vi "Update Vision Data.vi"(8 "error in (no error)":errorcluster, 10 "unsigned byte array":u8[](array[numeric]), 11 "Vision in":refnum<class "Vision.lvclass">) -> (0 "error out":errorcluster, 3 "Vision out":refnum<class "Vision.lvclass">)   [LabVIEW 2022 SP3, in "Vision.lvlib" / "Vision.lvclass"]
uses:
  Vision.lvclass
  Vision.lvclass/Vision.ctl
  Old vision/Decode SSL and Refree Wrapper Package Folder/Varint Decoder uint32.vi
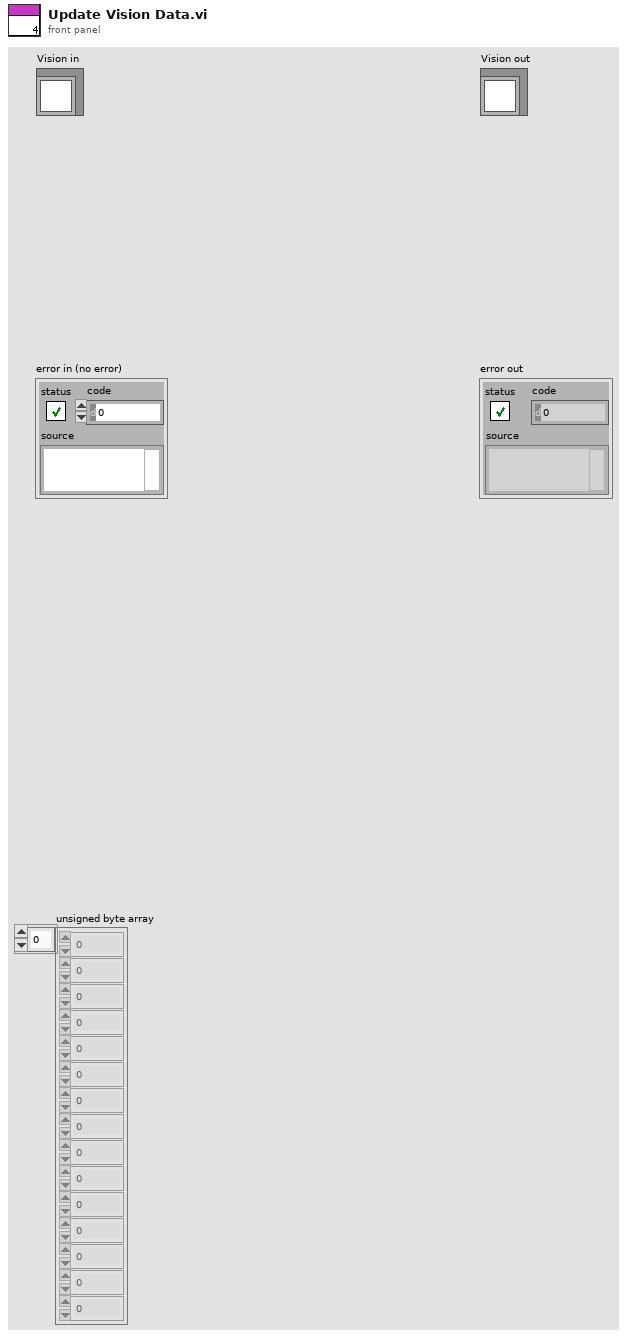
[diagram p1: front panel]
types:
  T1 = typedef "SSL Detection Frame.ctl" = cluster{"frame_number":u32, "t_capture":dbl, "t_sent":dbl, "camera_id":u32, "robots_yellow":T2[], "robots_blue":T2[], "balls":T4[], "Valid":bool, "Time Stamp":timestamp, "New":bool, "Initialized":bool}
  T2 = typedef "SSL Detection Robot.ctl" = cluster{"x":sgl, "robot_id":u32, "confidence":sgl, "y":sgl, "orientation":sgl, "pixel_x":sgl, "pixel_y":sgl, "height":sgl, "Valid":bool, "Time Stamp":timestamp, "x_k|k":T3, "Pk|k":T3, "Previous Time Stamp":timestamp, "R":T3, "vx":dbl, "vy":dbl, "vang":dbl}
  T3 = typedef "NI_Matrix.lvlib/RealMatrix.ctl" = dbl[][]
  T4 = typedef "SSL Detection Ball.ctl" = cluster{"x":sgl, "area":u32, "confidence":sgl, "y":sgl, "z":sgl, "pixel_x":sgl, "pixel_y":sgl, "Valid":bool, "Time Stamp":timestamp, "x_k|k":T3, "Pk|k":T3, "Id":u32, "Previous Time Stamp":timestamp, "R":T3, " vx":sgl, "vy":dbl, "vz":dbl, " ax":sgl, "ay":dbl, "az":dbl}
  T5 = typedef "SSL Geometry Camera Calibration.ctl" = cluster{"camera_id":u32, "focal_length":sgl, "principal_point_x":sgl, "principal_point_y":sgl, "distortion":sgl, "q0":sgl, "q1":sgl, "q2":sgl, "q3":sgl, "tx":sgl, "ty":sgl, "tz":sgl, "derived_camera_world_tx":sgl, "derived_camera_world_ty":sgl, "derived_camera_world_tz":sgl}
  T6 = cluster{"line_width":u32, "field_length":u32, "field_width":u32, "boundary_width":u32, "referee_width":u32, "goal_width":u32, "goal_depth":u32, "goal_wall_width":u32, "center_circle_radius":u32, "defense_radius":u32, "defense_stretch":u32, "free_kick_from_defense_dist":u32, "penalty_spot_from_field_line_dist":u32, "penalty_line_from_spot_dist":u32}
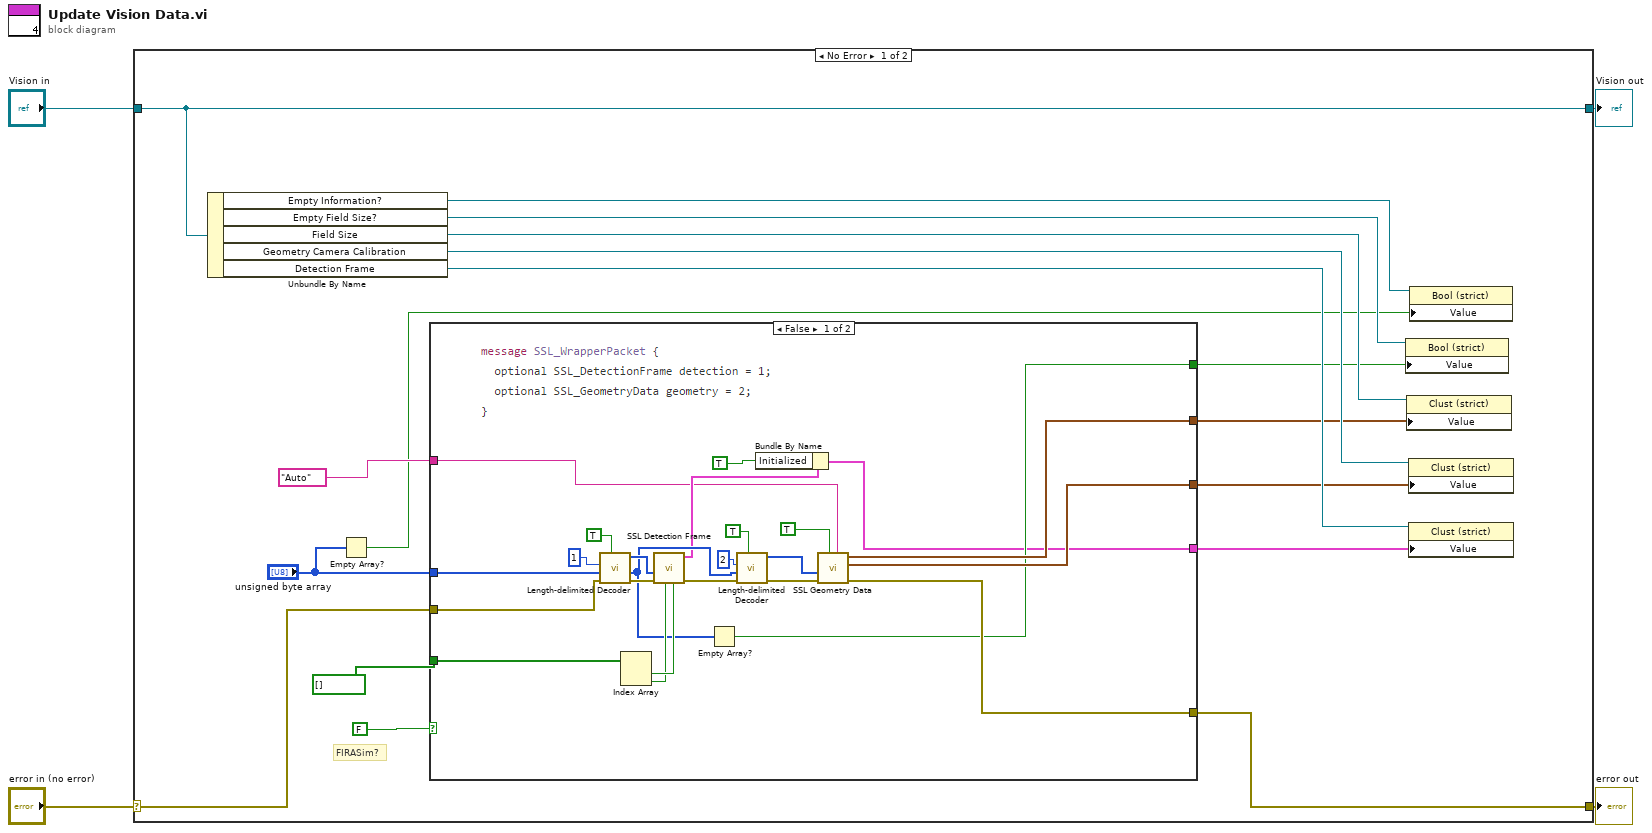
[diagram p0: block diagram]
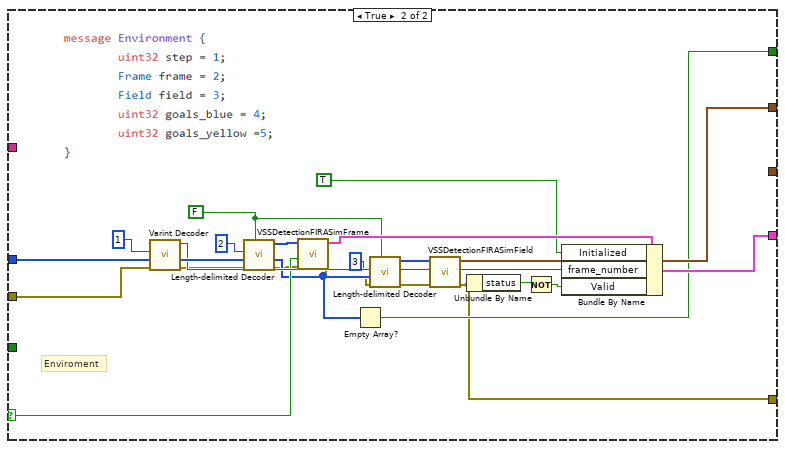
[diagram p2: hidden frame]
diagram:
  n1 = case shown="No Error" "error in (no error)" {
    selector: "error in (no error)" -> [w17 w71]
    tunnel: [w16 w71] -> w3
    tunnel: [w15 w70] -> w1
    tunnel: "Vision in" -> [w15 w70]
    frame No Error {
      # "FIRASim?"
      n2 = Unbundle By Name(w15) -> ("Empty Information?"=w14:refnum<vi>, "Empty Field Size?"=w13:refnum<vi>, "Field Size"=w12:refnum<vi>, "Geometry Camera Calibration"=w11:refnum<vi>, "Detection Frame"=w10:refnum<vi>)
      n3 = Empty Array?(array="unsigned byte array") -> (empty?=w9:bool)
      n4 = case shown="False" FALSE ("FIRASim?") {
        selector: FALSE ("FIRASim?") -> [_ w61]
        tunnel: [w45 w50] -> w16
        tunnel: bool[] [] ("Ignore left/rigth?") -> [w34 _]
        tunnel: [w31 w58] -> w7
        tunnel: [w30 _] -> w6
        tunnel: [w28 w56] -> w8
        tunnel: [w26 w62] -> w5
        tunnel: "unsigned byte array" -> [w24 w63]
        tunnel: w17 -> [w23 w53]
        tunnel: "Auto" ("Version") -> [w22 _]
        frame False {
          n5 = call "Length-delimited Decoder.vi"("Optional"=TRUE, "error in (no error)"=w23, "Array"=w24, "Key"=1) -> ("error out"=w37:errorcluster, "array w/ subset deleted"=w29:u8[], "Length-delimited"=w40:u8[])  [unwired: 4 in, 1 out]
          n6 = Index Array(array=w34) -> (element #1=w33:bool, element #2=w32:bool)  [unwired: 2 in]
          n7 = call "SSL Detection Frame.vi"("ignora esquerda?"=w33, "ignora direita?"=w32, "error in"=w37, "Array"=w40) -> ("error out"=w38:errorcluster, "Detection Frame"=w27:T1)  [unwired: 6 in]
          n8 = Empty Array?(array=w29) -> (empty?=w28:bool)
          n9 = call "Length-delimited Decoder.vi"("Optional"=TRUE, "error in (no error)"=w38, "Array"=w29, "Key"=2) -> ("error out"=w39:errorcluster, "Length-delimited"=w43:u8[])  [unwired: 4 in, 2 out]
          n10 = Bundle By Name(cluster=w27, "Initialized"=TRUE) -> (w26:T1)
          n11 = call "SSL Geometry Data.vi"("Version"=w22, "Optional"=TRUE, "error in"=w39, "Array"=w43) -> ("error out"=w45:errorcluster, "Geometry Camera Calibration"=w30:T5, "Field Size"=w31:T6)  [unwired: 5 in]
        }
        frame True {
          w46 = FALSE ("Optional")
          # "Enviroment"
          n12 = call-poly "Varint Decoder.vi"("error in (no error)"=w53, "Array"=w63, "Key"=1) -> ("error out"=w55:errorcluster, "array w/ subset deleted"=w68:u8[], "Varint"=w64:u32)  [unwired: 5 in, 1 out]
          n13 = call "Length-delimited Decoder.vi"("Optional"=w46, "error in (no error)"=w55, "Array"=w68, "Key"=2) -> ("error out"=w54:errorcluster, "array w/ subset deleted"=w57:u8[], "Length-delimited"=w66:u8[])  [unwired: 4 in, 1 out]
          n14 = call "VSSDetectionFIRASimFrame.vi"("error in (no error)"=w54, "FIRASim?"=w61, "Frame"=w66) -> ("error out"=w52:errorcluster, "Detection Frame out"=w65:T1)  [unwired: 7 in]
          n15 = Empty Array?(array=w57) -> (empty?=w56:bool)
          n16 = call "Length-delimited Decoder.vi"("Optional"=w46, "error in (no error)"=w52, "Array"=w57, "Key"=3) -> ("error out"=w51:errorcluster, "Length-delimited"=w59:u8[])  [unwired: 4 in, 2 out]
          n17 = call "VSSDetectionFIRASimField.vi"("error in (no error)"=w51, "Field"=w59) -> ("error out"=w50:errorcluster, "Field out"=w58:T6)  [unwired: 7 in, 1 out]
          n18 = Unbundle By Name(w50) -> ("status"=w49:bool)
          n19 = Not(x=w49) -> (.not. x?=w48:bool)
          n20 = Bundle By Name(cluster=w65, "Initialized"=TRUE, "frame_number"=w64, "Valid"=w48) -> (w62:T1)
        }
      }
      n21 = property class="Bool (strict)"(reference=w13, "Value"=w8) -> ()  [unwired: 1 in, 2 out]
      n22 = property class="Clust (strict)"(reference=w12, "Value"=w7) -> ()  [unwired: 1 in, 2 out]
      n23 = property class="Clust (strict)"(reference=w11, "Value"=w6) -> ()  [unwired: 1 in, 2 out]
      n24 = property class="Clust (strict)"(reference=w10, "Value"=w5) -> ()  [unwired: 1 in, 2 out]
      n25 = property class="Bool (strict)"(reference=w14, "Value"=w9) -> ()  [unwired: 1 in, 2 out]
    }
    frame Error {
    }
  }
  "error out" <- w3
  "Vision out" <- w1
